vi "Get and Flatten.vi"(8 "error in (no error)":errorcluster, 11 "CAN Data in":refnum<class "CAN Data.lvclass">) -> (0 "error out":errorcluster, 2 "Flattened data string":string, 3 "CAN Data out":refnum<class "CAN Data.lvclass">)   [LabVIEW 2021, in "BS120x Driver.lvlib" / "Data Classes.lvlib" / "CAN Data.lvclass"]
uses:
  CAN Data.lvclass
  CAN Data.lvclass/CAN Data.ctl
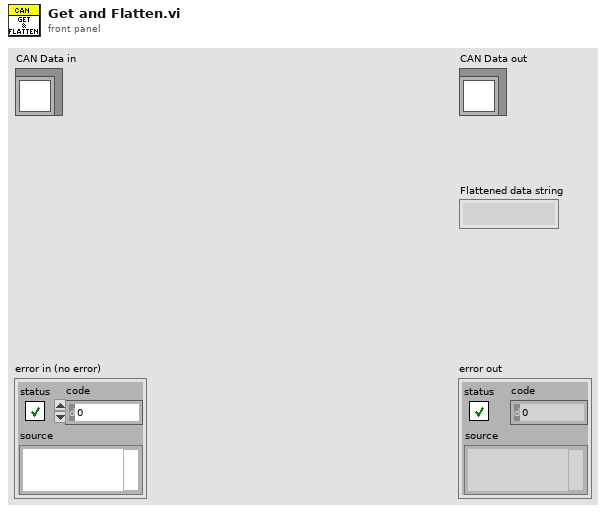
[diagram p1: front panel]
types:
  T1 = cluster{"identifier":u32, "extended?":bool, "type":enum8{"CAN Data", "CAN Remote"}, "payload":u8[]}[]
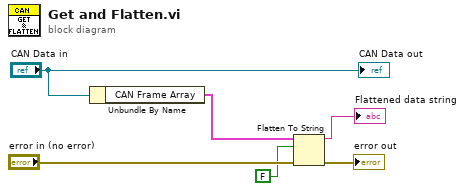
[diagram p0: block diagram]
diagram:
  n1 = Unbundle By Name("CAN Data in") -> ("CAN Frame Array"=w2:T1)
  n2 = Flatten To String(anything=w2, prepend array or string size? (T)=FALSE, error in (no error)="error in (no error)") -> (data string=→"Flattened data string":string, error out=→"error out":errorcluster)  [unwired: 2 out]
  "CAN Data out" <- "CAN Data in"
